vi "Q_Get Type distances for Athlete.vi"(8 "error in (no error)":errorcluster, 10 "Alias":string, 11 "Data Manager in":refnum<class "Data Manager.lvclass">) -> (0 "error out":errorcluster, 1 "Array":dbl[](array[numeric]), 2 "output cluster":cluster{dbl, dbl, dbl}, 3 "Data Manager out":refnum<class "Data Manager.lvclass">)   [LabVIEW 2020, in "Data Manager.lvclass"]
uses:
  Data Manager.lvclass
  Data Manager.lvclass/Data Manager.ctl
  <vilib>/drjdpowell/SQLite Library/SQL Connection/Execute SQL (Single DBL).vi
  <vilib>/drjdpowell/SQLite Library/SQLite.lvlib
  <vilib>/drjdpowell/SQLite Library/SQL Connection/Connection.lvclass
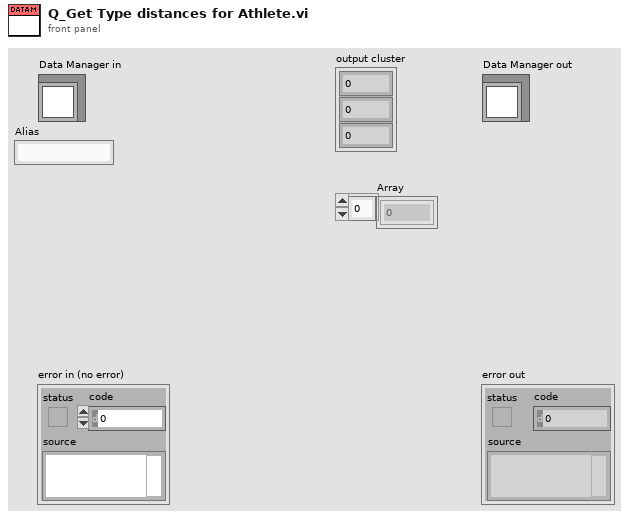
[diagram p1: front panel]
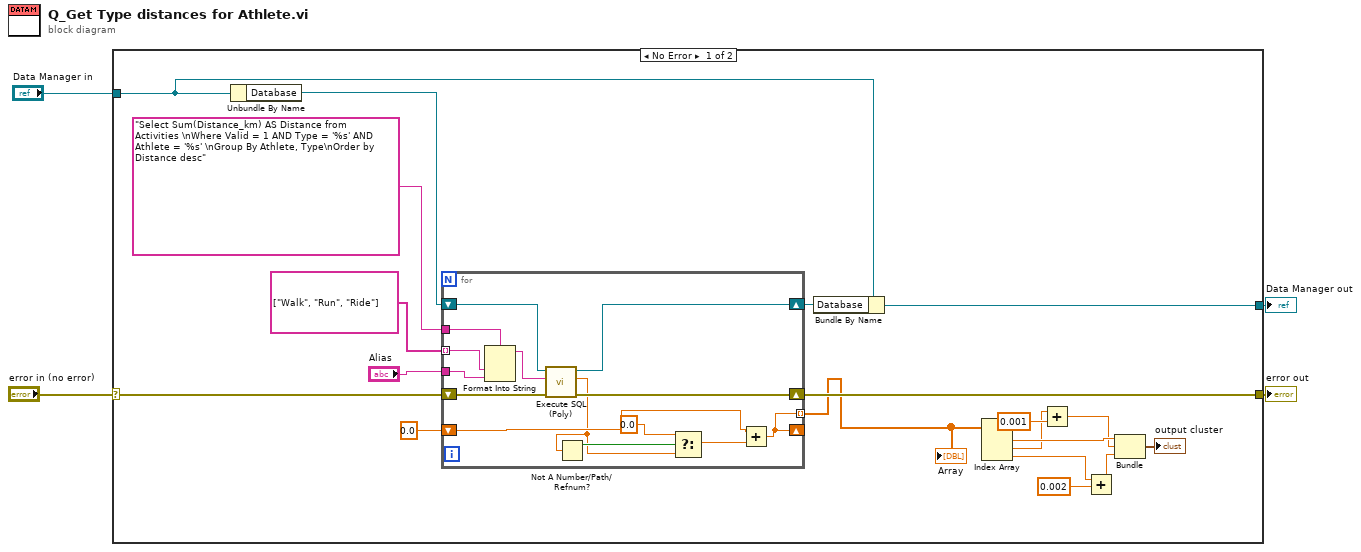
[diagram p0: block diagram]
diagram:
  n1 = case shown="No Error" "error in (no error)" {
    selector: "error in (no error)" -> [w19 w39]
    tunnel: [w18 w39] -> w3
    tunnel: [w21 w38] -> w1
    tunnel: "Data Manager in" -> [w22 w38]
    frame No Error {
      n2 = Unbundle By Name(w22) -> ("Database"=w23:refnum<class "Connection.lvclass">)
      n3 = for {
        tunnel: "Select Sum(Distance_km) AS Distance from Activities \nWhere Valid = 1 AND Type = '%s' AND Athlete = '%s' \nGroup By Athlete, Type\nOrder by Distance desc" ("SQL") -> [w33]
        shift-right: [w36] -> w20
        shift-left: w23 -> [w37]
        shift-right: [w34] -> w18
        shift-left: w19 -> [w35]
        tunnel: string[] ["Walk", "Run", "Ride"] -> [w31] mode=indexing
        tunnel: "Alias" -> [w30]
        shift-right: [w26] -> _
        shift-left: 0.0 -> [w25]
        tunnel: [w26] -> w13 mode=indexing
        n4 = Format Into String(format string=w33, w31, w30) -> (resulting string=w32:string)  [unwired: 2 in, 1 out]
        n5 = call-poly <vilib>:"Execute SQL (Poly).vi"("error in (no error)"=w35, "SQL"=w32, "SQLite Connection in"=w37) -> ("error out"=w34:errorcluster, "Result"=w24:dbl, "SQLite Connection"=w36:refnum<class "Connection.lvclass">)  [unwired: 6 in]
        n6 = Not A Number/Path/Refnum?(number/path/refnum=w24) -> (NaN/Path/Refnum?=w29:bool)
        n7 = Select(t=0.0, s=w29, f=w24) -> (s? t:f=w27:dbl)
        n8 = Add(x=w25, y=w27) -> (x+y=w26:dbl)
      }
      "Array" <- w13
      n9 = Bundle By Name(cluster=w22, "Database"=w20) -> (w21:refnum<class "Data Manager.lvclass">)
      n10 = Index Array(array=w13) -> (element #1=w11:dbl, element #2=w8:dbl, element #3=w7:dbl)  [unwired: 3 in]
      n11 = Add(x=w8, y=0.001) -> (x+y=w9:dbl)
      n12 = Add(x=w7, y=0.002) -> (x+y=w6:dbl)
      n13 = Bundle(w11, w9, w6) -> (→"output cluster":cluster{dbl, dbl, dbl})  [unwired: 1 in]
    }
    frame Error {
    }
  }
  "error out" <- w3
  "Data Manager out" <- w1
